vi "singleTrial_noReturn_multiPlatform.vi"() -> ()   [LabVIEW 2017]
uses:
  <vilib>/Utility/file.llb/Read Delimited Spreadsheet (DBL).vi
  <vilib>/Utility/file.llb/Write Delimited Spreadsheet (I64).vi
panel:
  in  "Max number of platforms to \npick":i32=2
  in  "difficulty":string(combo)="1"
  in  "Maze rotation":string(combo)="clockwise"
  in  "Choice/goal platforms up or down?":string(combo)="up"
  in  "Rat ID":string
  out "choices":i32[][](array[numeric])
  in  "Goal \nplatform":i32
  in  "start platform":i32
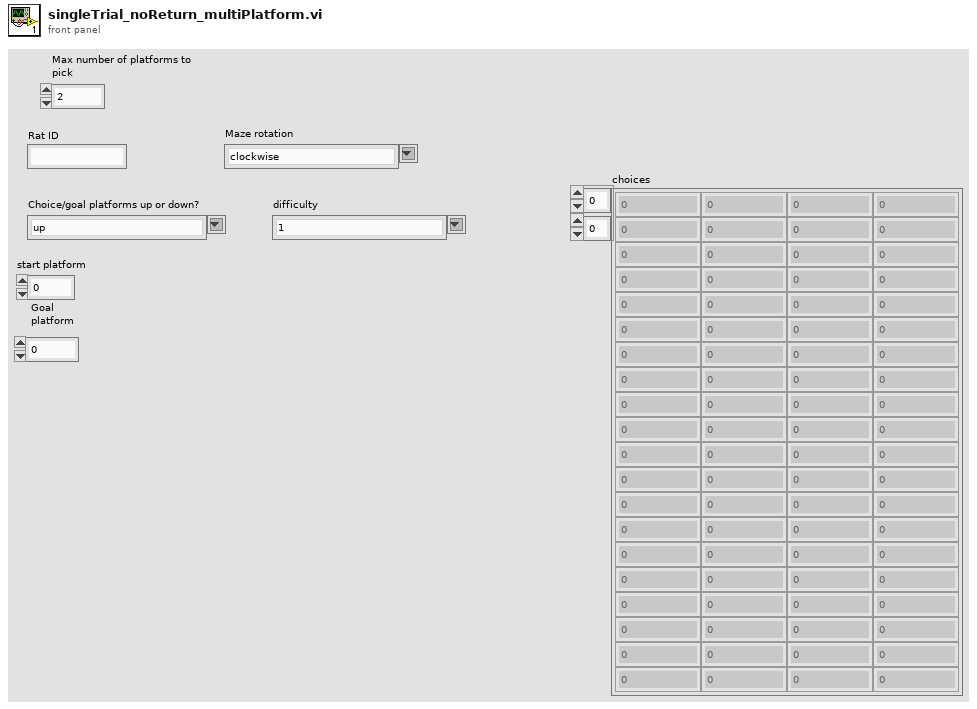
[diagram p1: front panel]
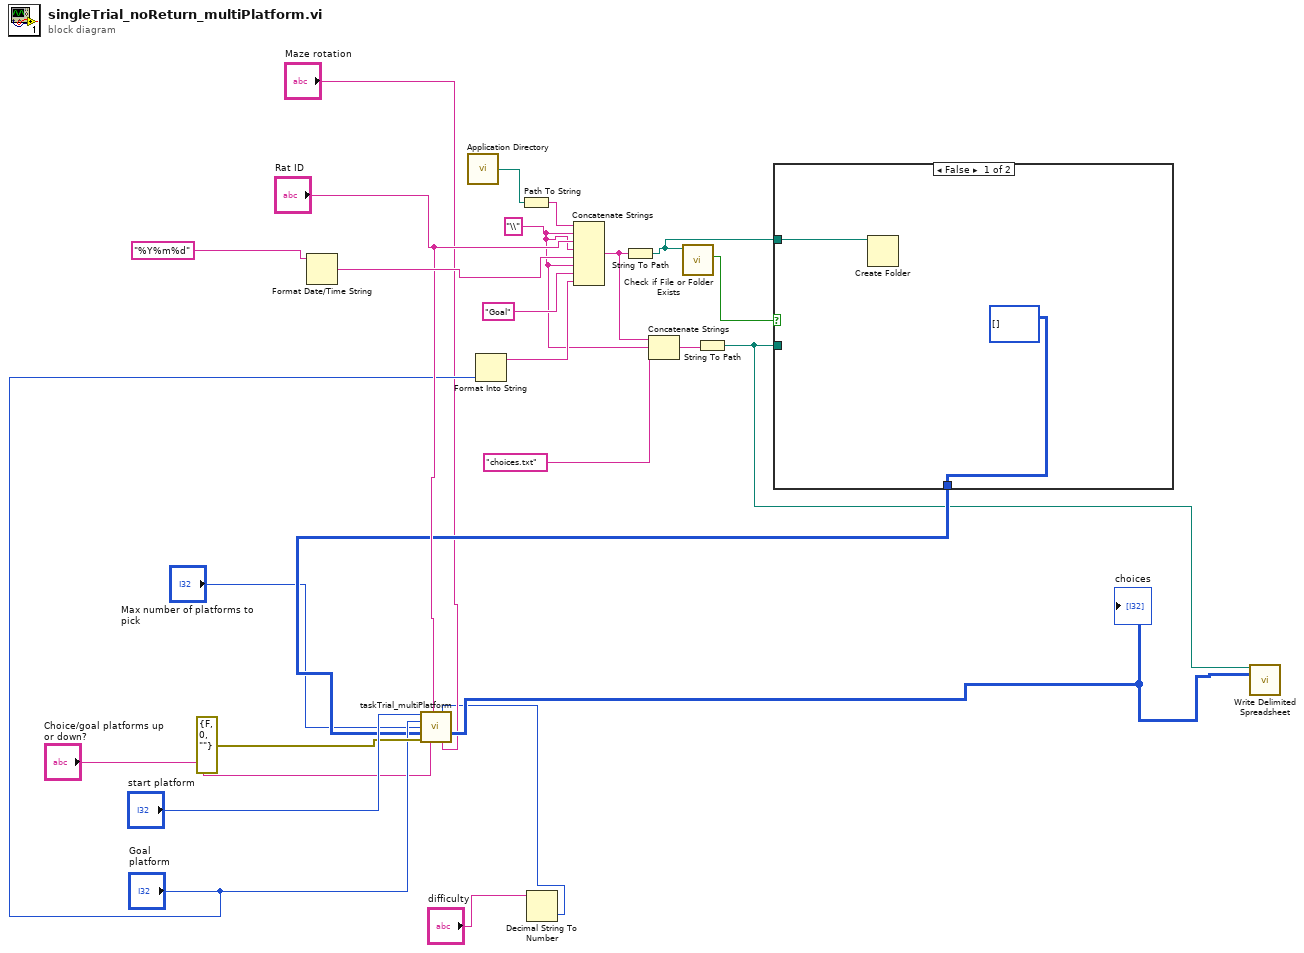
[diagram p0: block diagram]
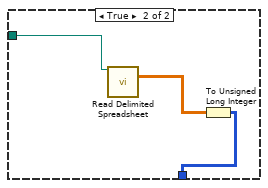
[diagram p2: hidden frame]
diagram:
  w13 = "\\" ("string")
  n1 = Format Date/Time String(time format string (%c)="%Y%m%d" ("time string")) -> (date/time string=w20:string)  [unwired: 2 in]
  n2 = call <vilib>:"Application Directory.vi"() -> ("Application Directory"=w19:path)
  n3 = Format Into String("Goal \nplatform") -> (resulting string=w15:string)  [unwired: 3 in, 1 out]
  n4 = Path To String(path=w19) -> (string=w22:string)
  n5 = Decimal String To Number(string="difficulty") -> (number=w2:i32)  [unwired: 2 in, 1 out]
  n6 = Concatenate Strings(w22, w13, "Rat ID", w13, w20, w13, "Goal" ("string"), w15) -> (w12:string)
  n7 = String To Path(string=w12) -> (path=w8:path)
  n8 = Concatenate Strings(w12, w13, "choices.txt" ("string")) -> (w10:string)
  n9 = call <vilib>:"Check if File or Folder Exists.vi"("path"=w8) -> ("file or folder exists?"=w14:bool)  [unwired: 8 in, 2 out]
  n10 = String To Path(string=w10) -> (path=w7:path)
  n11 = case shown="False" w14 {
    tunnel: w7 -> [_ w29]
    tunnel: [i32[][] [] ("previousChoices") w27] -> w9
    tunnel: w8 -> [w25 _]
    frame False {
      n12 = Create Folder(path (use dialog)=w25) -> ()  [unwired: 2 in, 3 out]
    }
    frame True {
      n13 = call-poly <vilib>:"Read Delimited Spreadsheet.vi"("file path (dialog if empty)"=w29) -> ("all rows"=w28:dbl[][])  [unwired: 9 in, 5 out]
      n14 = To Unsigned Long Integer(number=w28) -> (unsigned 32bit integer=w27:u32[][])
    }
  }
  n15 = call "taskTrial_multiPlatform.vi"("Start \nplatform"="start platform", "Rat ID"="Rat ID", "difficulty"=w2, "Goal \nplatform"="Goal \nplatform", "Max number of platforms to \npick"="Max number of platforms to \npick", "previousChoices"=w9, "error in (no error)"=errorcluster {"status"=FALSE, "code"=0, "source"=""}, "up or down"="Choice/goal platforms up or down?", "mazeDirection"="Maze rotation") -> ("previousChoices updated"=w5:i32[][])  [unwired: 4 in, 2 out]
  "choices" <- w5
  n16 = call-poly <vilib>:"Write Delimited Spreadsheet.vi"("file path (dialog if empty)"=w7, "2D data"=w5) -> ()  [unwired: 12 in, 2 out]
